vi "Finish.vi"(8 "error in (no error)":errorcluster, 11 "XBoxController in":refnum<class "XBoxController.lvclass">) -> (0 "error out":errorcluster, 3 "XBoxController out":refnum<class "XBoxController.lvclass">)   [LabVIEW 2013, in "XBoxController.lvclass"]
uses:
  XBoxController.lvclass
  System/System.lvclass
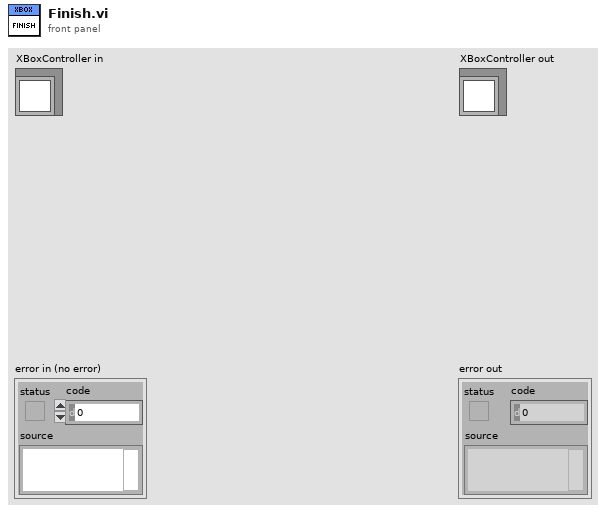
[diagram p1: front panel]
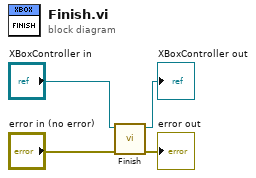
[diagram p0: block diagram]
diagram:
  n1 = call-parent "Finish.vi"("error in (no error)"="error in (no error)", "System in"="XBoxController in") -> ("error out"=→"error out":errorcluster, "System out"=→"XBoxController out":refnum<class "XBoxController.lvclass">)  [unwired: 8 in]
